vi "CoboltLaser_CurrentSetpointGet.vi"(6 "CurrentModLow":bool, 8 "ErrorIn":errorcluster, 9 "Mode":T1 caption="Laser Mode", 10 "CheckResponse":bool=TRUE, 11 "ComPort":refnum<visa-resource-name>) -> (0 "ErrorOut":errorcluster, 1 "Response":string, 2 "LaserCurrent":dbl format="%.3g", 3 "ComPortOut":refnum<visa-resource-name>, 4 "ResponseOK":bool)   [LabVIEW 2019]
doc: "Use this template to build a VI to use as a subVI."
uses:
  Programmes Labview/LabscanV1A/DevicesClass/InstrumentsClass/CoboltMLD/CoboltModes.ctl
panel:
  # "(mA)"
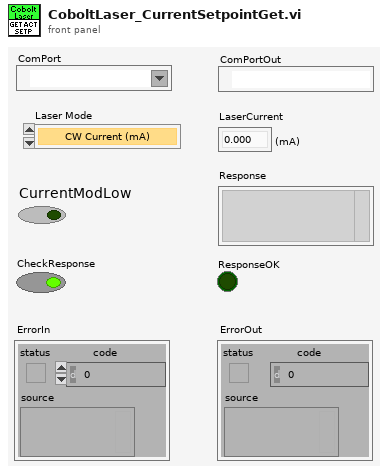
[diagram p1: front panel]
types:
  T1 = typedef "CoboltModes.ctl" = enum16{"CW Current (mA)", "CW Power (mW)", "Current Mod. (mA)", "Power Mod. (mA)"}
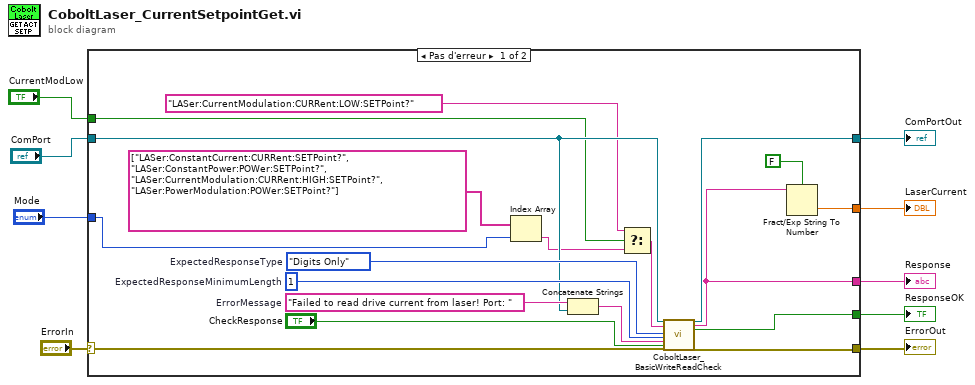
[diagram p0: block diagram]
diagram:
  n1 = case shown="Pas d'erreur" "ErrorIn" {
    selector: "ErrorIn" -> [w28 w30]
    tunnel: [w27 w30] -> w8
    tunnel: "ComPort" -> [w21 w29]
    tunnel: [w20 w29] -> w6
    tunnel: [w18 _] -> w5
    tunnel: [w17 _] -> w4
    tunnel: [w16 _] -> w3
    tunnel: "Mode" -> [w14 _]
    tunnel: "CurrentModLow" -> [w10 _]
    frame No Error {
      w25 = 1  # ExpectedResponseMinimumLength
      w26 = enum16{"Any", "Digits Only", "Non-Digits Only"}."Digits Only"  # ExpectedResponseType
      w23 = "Failed to read drive current from laser! Port: "  # ErrorMessage
      n2 = Index Array(array=string[] ["LASer:ConstantCurrent:CURRent:SETPoint?", "LASer:ConstantPower:POWer:SETPoint?", "LASer:CurrentModulation:CURRent:HIGH:SETPoint?", "LASer:PowerModulation:POWer:SETPoint?"] ("tableau ajouté"), index=w14) -> (element=w12:string)
      n3 = Concatenate Strings(w23, w21) -> (w22:string)
      n4 = Select(t="LASer:CurrentModulation:CURRent:LOW:SETPoint?" ("Command"), s=w10, f=w12) -> (s? t:f=w13:string)
      n5 = call <userlib>:"CoboltLaser_BasicWriteReadCheck.vi"("ComPort"=w21, "Command"=w13, "ExpectedResponseType"=w26, "ExpectedResponseMinimumLength"=w25, "ErrorMessage"=w22, "GenerateError"="CheckResponse", "error in (no error)"=w28) -> ("ComPortOut"=w20:refnum<visa-resource-name>, "Response"=w17:string, "ResponseOK"=w16:bool, "error out"=w27:errorcluster)  [unwired: 17 in]
      n6 = Fract/Exp String To Number(use system decimal point (T)=FALSE, string=w17) -> (number=w18:dbl)  [unwired: 2 in, 1 out]
    }
    frame Error {
    }
  }
  "ErrorOut" <- w8
  "ComPortOut" <- w6
  "Response" <- w4
  "ResponseOK" <- w3
  "LaserCurrent" <- w5
